vi "Test Write 2.vi"() -> ()   [LabVIEW 2014, in "Arduino SoftwareSerial Wrapper.lvlib"]
uses:
  Arduino SoftwareSerial Wrapper.lvlib
panel:
  out "Bytes to read":u16
  out "Error Out":errorcluster
  in  "Error In":errorcluster
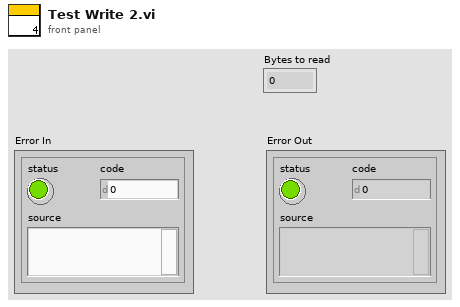
[diagram p1: front panel]
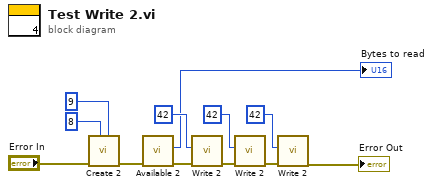
[diagram p0: block diagram]
diagram:
  n1 = call "Create 2.vi"("arduino RX pin"=u8 9 ("RX pin"), "arduino TX pin"=u8 8 ("RX pin"), "Error In"="Error In") -> ("Error Out"=w9:errorcluster)  [unwired: 8 in]
  n2 = call "Available 2.vi"("Error In"=w9) -> ("Error Out"=w8:errorcluster, "Bytes to read"=→"Bytes to read":u16)  [unwired: 9 in]
  n3 = call "Write 2.vi"("Error In"=w8, "Char to write"=u8 42) -> ("Error Out"=w4:errorcluster)  [unwired: 9 in]
  n4 = call "Write 2.vi"("Error In"=w4, "Char to write"=u8 42) -> ("Error Out"=w3:errorcluster)  [unwired: 9 in]
  n5 = call "Write 2.vi"("Error In"=w3, "Char to write"=u8 42) -> ("Error Out"=→"Error Out":errorcluster)  [unwired: 9 in]
